vi "Pockels Cal-Exctract cal header.vi"(11 "Pockels Cal table (full)":string[][](array[string])) -> (3 "Cal data header":string[](array[string]))   [LabVIEW 2017]
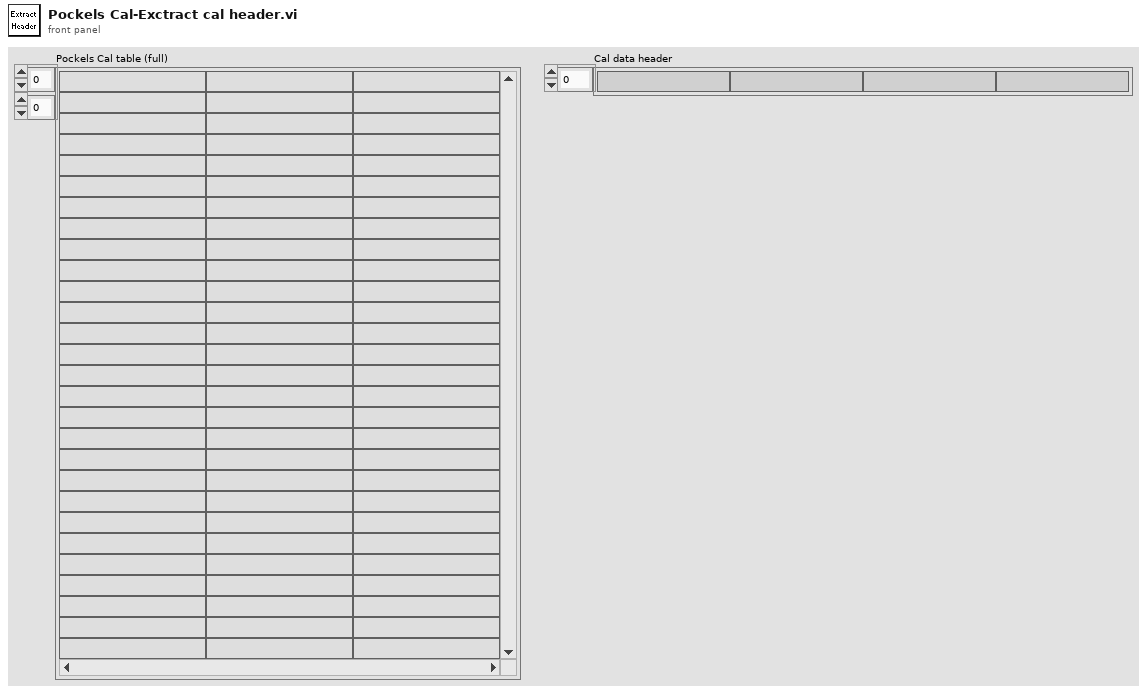
[diagram p1: front panel]
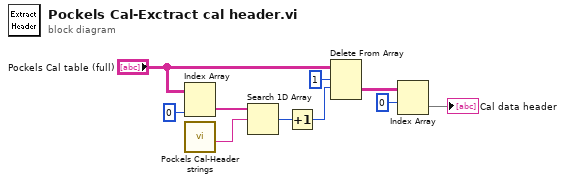
[diagram p0: block diagram]
diagram:
  n1 = Index Array(array="Pockels Cal table (full)", index (col)=0 ("disabled index (col)")) -> (element=w5:string[])  [unwired: 1 in]
  n2 = call "Pockels Cal-Header strings.vi"() -> ("Cal data header string"=w7:string)  [unwired: 9 in, 2 out]
  n3 = Search 1D Array(1D array=w5, element=w7) -> (index of element=w8:i32)  [unwired: 1 in]
  n4 = Increment(x=w8) -> (x+1=w9:i32)
  n5 = Delete From Array "Delete From Array"(array="Pockels Cal table (full)", length=1, index (row)=w9) -> (deleted portion=w3:string[][])  [unwired: 1 in, 1 out]
  n6 = Index Array "Index Array"(array=w3, index (row)=0) -> (element=→"Cal data header":string[])  [unwired: 1 in]
